vi "rethinkdb_hashlib_scram_client_proof.vi"(5 "client_first_message":string, 6 "password":string, 7 "server_first_message":string, 9 "i":i32, 10 "s":string, 11 "r":string) -> (3 "client_final_msg":string)   [LabVIEW 2017]
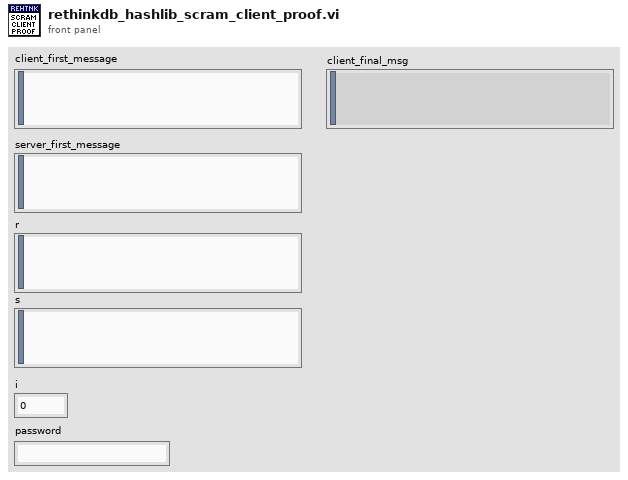
[diagram p1: front panel]
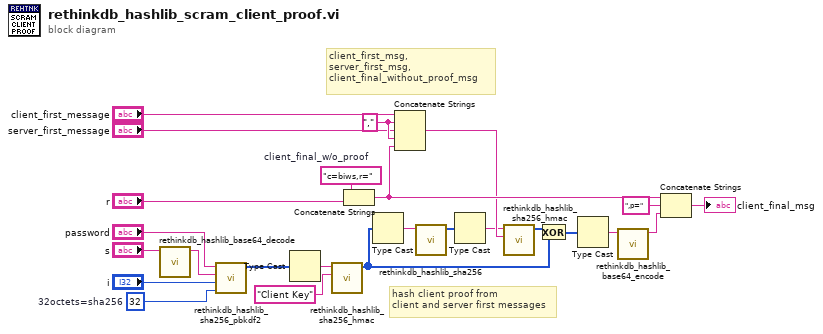
[diagram p0: block diagram]
diagram:
  w18 = "," ("string")
  w16 = "c=biws,r="  # client_final_w/o_proof
  w8 = 32  # 32octets=sha256
  # "hash client proof from \nclient and server first messages"
  # "client_first_msg,\nserver_first_msg,\nclient_final_without_proof_msg"
  n1 = call "rethinkdb_hashlib_base64_decode.vi"("base64"="s") -> ("string"=w1:string)  [unwired: 10 in]
  n2 = call "rethinkdb_hashlib_sha256_pbkdf2.vi"("dkLen (32octets=sha256)"=w8, "iterations"="i", "salt"=w1, "password"="password") -> ("sha-256"=w9:u32[])  [unwired: 7 in]
  n3 = Type Cast(x=w9) -> (*(type *) &x=w11:string)  [unwired: 1 in]
  n4 = call "rethinkdb_hashlib_sha256_hmac.vi"("data"="Client Key" ("key"), "key"=w11) -> ("sha256"=w5:u32[])  [unwired: 9 in]
  n5 = Concatenate Strings(w16, "r") -> (w22:string)
  n6 = Type Cast(x=w5) -> (*(type *) &x=w2:string)  [unwired: 1 in]
  n7 = Concatenate Strings("client_first_message", w18, "server_first_message", w18, w22) -> (w19:string)
  n8 = call "rethinkdb_hashlib_sha256.vi"("data"=w2) -> ("sha256"=w3:u32[])  [unwired: 10 in]
  n9 = Type Cast(x=w3) -> (*(type *) &x=w10:string)  [unwired: 1 in]
  n10 = call "rethinkdb_hashlib_sha256_hmac.vi"("data"=w19, "key"=w10) -> ("sha256"=w4:u32[])  [unwired: 9 in]
  n11 = Exclusive Or(1:w5, 2:w4) -> (0:w6:u32[])
  n12 = Type Cast(x=w6) -> (*(type *) &x=w7:string)  [unwired: 1 in]
  n13 = call "rethinkdb_hashlib_base64_encode.vi"("string"=w7) -> ("base64"=w24:string)  [unwired: 10 in]
  n14 = Concatenate Strings(w22, ",p=", w24) -> (→"client_final_msg":string)
